vi "Demo1 (FPGA).vi"   [LabVIEW 2023]
uses:
  <vilib>/eio/EIONode/EIONode.xnode
  Instance           1 20Saved   Demo1 (FPGA) .vi
  <vilib>/rvi/eio/common/nirviEmuTemplateMethod_errors.vi
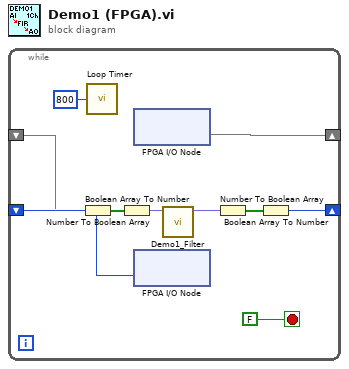
[diagram p0: block diagram]
diagram:
  n1 = while {
    shift-right: [w10] -> _
    shift-left: _ -> [w5]
    shift-right: [w1] -> _
    shift-left: _ -> [w8]
    stop <- FALSE stop-if-true
    n2 = Number To Boolean Array(number=w5) -> (Boolean array=w4:bool[])
    n3 = call "Loop Timer"("Count(Ticks)"=u32 800) -> ()  [unwired: 1 out]
    n4 = Boolean Array To Number(Boolean array=w4) -> (number=w3:fxp<+/-,16,1>)
    n5 = xnode "FPGA I/O Node"() -> ("AI0"=w10)  [unwired: 1 in, 1 out]
    n6 = xnode "FPGA I/O Node"("AO0"=w8) -> ()  [unwired: 1 in, 1 out]
    n7 = call "Demo1_Filter.vi"("input data"=w3) -> ("output data"=w9:fxp<+/-,16,2>)  [unwired: 1 in, 9 out]
    n8 = Number To Boolean Array(number=w9) -> (Boolean array=w2:bool[])
    n9 = Boolean Array To Number(Boolean array=w2) -> (number=w1:i16)
  }
